vi "因式分解.vi"() -> ()   [LabVIEW 2013]
panel:
  in  "输入":i32
  in  "因数":i32=2
  out "分解":i32[](array[numeric])
  out "中间变量":i32
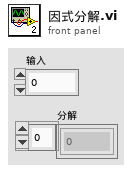
[diagram p1: front panel]
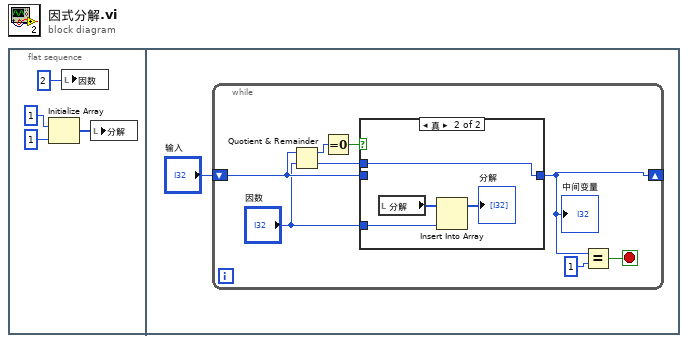
[diagram p0: block diagram]
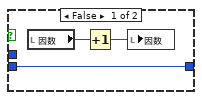
[diagram p2: hidden frame]
diagram:
  n1 = flat-sequence {
    frame #0 {
      n2 = Initialize Array(1 ("元素"), 1 ("维数大小")) -> (w1:i32[])
      n3 = local write "因数"(2 ("因数")) -> ()
      n4 = local write "分解"(w1) -> ()
    }
    frame #1 {
      n5 = while {
        shift-right: [w10] -> _
        shift-left: "输入" -> [w11]
        stop <- w8 stop-if-true
        n6 = Quotient & Remainder(x=w11, y="因数") -> (x-y*floor(x/y)=w13:i32, floor(x/y)=w12:i32)
        n7 = Equal To 0?(x=w13) -> (x = 0?=w6:bool)
        n8 = case shown="真" w6 {
          tunnel: [w16 w20] -> w10
          tunnel: w12 -> [_ w20]
          tunnel: w11 -> [w16 _]
          tunnel: "因数" -> [_ w18]
          frame False {
            n9 = local read "因数"() -> (w15:i32)
            n10 = Increment(x=w15) -> (x+1=w14:i32)
            n11 = local write "因数"(w14) -> ()
          }
          frame True {
            n12 = local read "分解"() -> (w19:i32[])
            n13 = Insert Into Array(array=w19, new element=w18) -> (→"分解":i32[])  [unwired: 1 in]
          }
        }
        "中间变量" <- w10
        n14 = Equal?(x=w10, y=1) -> (x = y?=w8:bool)
      }
    }
  }
